vi "Time.vi"(6 "Set/Check (F: Set)":bool, 7 "Date/Time/Both (0:Date)":enum16{"Date", "Time", "Date and Time"}(ring), 8 "error in (no error)":errorcluster, 9 "Time (0\\0\\0.0)":cluster{"Second":dbl, "Minute":u16, "Hour":u16} {"Hour" max=24; "Minute" max=59; "Second" min=0.0 max=60.0 format="%.3f"}, 10 "Date (1\\1\\1997)":cluster{"Day":u16, "Month":u16, "Year":u16}={"Day"=1, "Month"=0, "Year"=1997} {"Year" min=1997; "Month" items=["January", "February", "March", "April", "May", "June", "July", "August", "September", "October", "November", "December"]; "Day" min=1 max=31}, 11 "VISA Resource Name":refnum<visa-resource-name>) -> (0 "error out":errorcluster, 2 "read buffer":string, 3 "VISA Resource Name Out":refnum<visa-resource-name>)   [LabVIEW 2016, in "Agilent 34970.lvlib"]
doc: "This VI allows you to set the date and time on the instrument. Choose whether you wish to set or check the date (default), time, or both date and time."
uses:
  Agilent 34970.lvlib
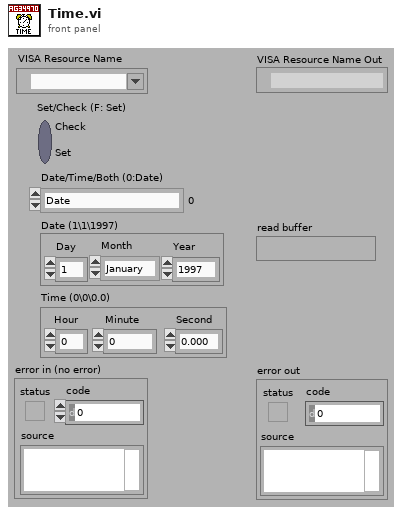
[diagram p1: front panel]
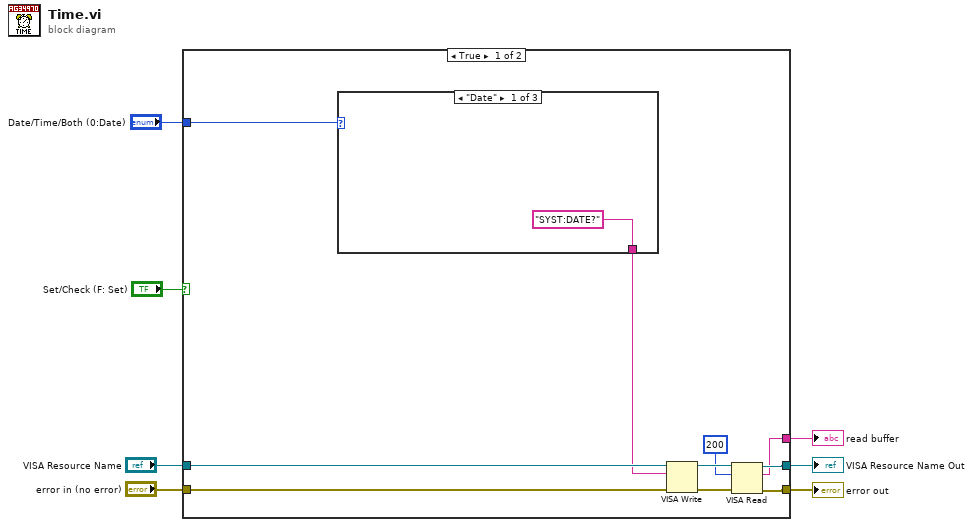
[diagram p0: block diagram]
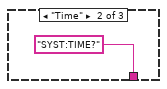
[diagram p2: hidden frame]
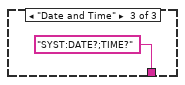
[diagram p3: hidden frame]
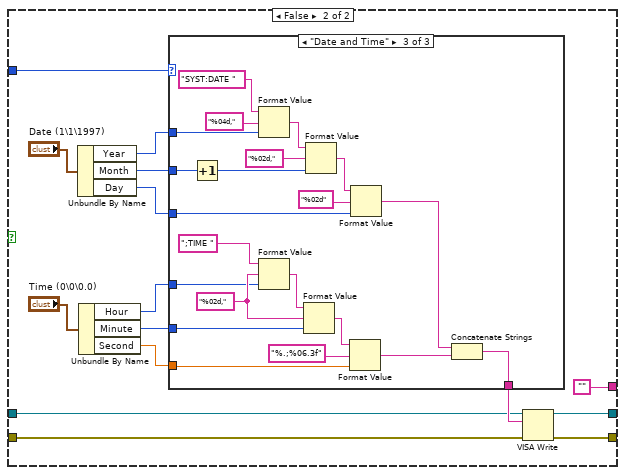
[diagram p4: hidden frame]
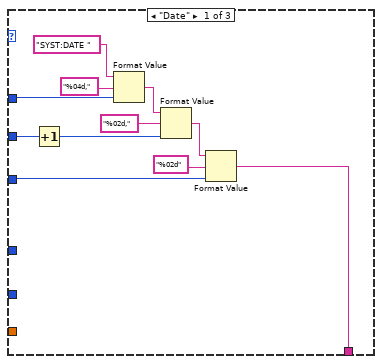
[diagram p5: hidden frame]
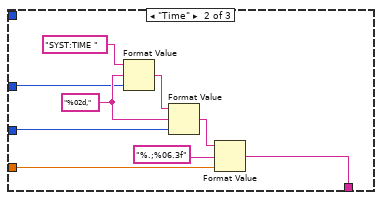
[diagram p6: hidden frame]
diagram:
  n1 = case shown="True" "Set/Check (F: Set)" {
    tunnel: "Date/Time/Both (0:Date)" -> [w17 w35]
    tunnel: "VISA Resource Name" -> [w16 w25]
    tunnel: "error in (no error)" -> [w15 w24]
    tunnel: [w11 w23] -> w3
    tunnel: [w10 w22] -> w2
    tunnel: [w9 ""] -> w1
    frame True {
      n2 = case shown="\"Date\"" w17 {
        tunnel: ["SYST:DATE?" "SYST:TIME?" "SYST:DATE?;TIME?"] -> w8
        frame "Date" {
        }
        frame "Time" {
        }
        frame "Date and Time" {
        }
      }
      n3 = VISA Write(VISA resource name=w16, write buffer=w8, error in (no error)=w15) -> (VISA resource name out=w14:refnum<visa-resource-name>, error out=w13:errorcluster)  [unwired: 1 out]
      n4 = VISA Read(VISA resource name=w14, byte count=u32 200, error in (no error)=w13) -> (VISA resource name out=w11:refnum<visa-resource-name>, read buffer=w9:string, error out=w10:errorcluster)  [unwired: 1 out]
    }
    frame False {
      n5 = Unbundle By Name("Date (1\\1\\1997)") -> ("Year"=w32:u16, "Month"=w33:u16, "Day"=w34:u16)
      n6 = Unbundle By Name("Time (0\\0\\0.0)") -> ("Hour"=w30:u16, "Minute"=w29:u16, "Second"=w28:dbl)
      n7 = case shown="\"Date and Time\"" w35 {
        tunnel: [w38 w47 w64] -> w26
        tunnel: w32 -> [w40 _ w63]
        tunnel: w33 -> [w37 _ w58]
        tunnel: w34 -> [w39 _ w62]
        tunnel: w29 -> [_ w49 w61]
        tunnel: w30 -> [_ w50 w60]
        tunnel: w28 -> [_ w48 w59]
        frame "Date" {
          n8 = Increment(x=w37) -> (x+1=w36:u16)
          n9 = Format Value(string ("")="SYST:DATE ", format string="%04d,", value (0)=w40) -> (output string=w43:string)
          n10 = Format Value(string ("")=w43, format string="%02d,", value (0)=w36) -> (output string=w44:string)
          n11 = Format Value(string ("")=w44, format string="%02d", value (0)=w39) -> (output string=w38:string)
        }
        frame "Time" {
          w54 = "%02d," ("format string")
          n12 = Format Value(string ("")="SYST:TIME ", format string=w54, value (0)=w50) -> (output string=w51:string)
          n13 = Format Value(string ("")=w51, format string=w54, value (0)=w49) -> (output string=w52:string)
          n14 = Format Value(string ("")=w52, format string="%.;%06.3f", value (0)=w48) -> (output string=w47:string)
        }
        frame "Date and Time" {
          w73 = "%02d," ("format string")
          n15 = Increment(x=w58) -> (x+1=w57:u16)
          n16 = Format Value(string ("")="SYST:DATE ", format string="%04d,", value (0)=w63) -> (output string=w68:string)
          n17 = Format Value(string ("")=";TIME ", format string=w73, value (0)=w60) -> (output string=w70:string)
          n18 = Format Value(string ("")=w70, format string=w73, value (0)=w61) -> (output string=w71:string)
          n19 = Format Value(string ("")=w68, format string="%02d,", value (0)=w57) -> (output string=w69:string)
          n20 = Format Value(string ("")=w71, format string="%.;%06.3f", value (0)=w59) -> (output string=w65:string)
          n21 = Format Value(string ("")=w69, format string="%02d", value (0)=w62) -> (output string=w56:string)
          n22 = Concatenate Strings(w56, w65) -> (w64:string)
        }
      }
      n23 = VISA Write(VISA resource name=w25, write buffer=w26, error in (no error)=w24) -> (VISA resource name out=w23:refnum<visa-resource-name>, error out=w22:errorcluster)  [unwired: 1 out]
    }
  }
  "VISA Resource Name Out" <- w3
  "error out" <- w2
  "read buffer" <- w1
